vi "Get.vi"(6 "abort (F)":bool, 11 "TagData in":refnum<class "TagData.lvclass">) -> (0 "element":cluster{timestamp[], dbl[]}[](array[cluster]), 1 "sequence":u64, 2 "update":refnum<k4>, 3 "TagData out":refnum<class "TagData.lvclass">, 4 "aborted?":bool)   [LabVIEW 2020, in "Tag-a[.](c(a[.](stamp),a[.](dbl))).lvlib" / "TagData.lvclass"]
uses:
  <extravilib>/ChannelInstances/Tag-a[.](c(a[.](stamp),a[.](dbl)))/TagData.lvclass
  <extravilib>/ChannelInstances/Tag-a[.](c(a[.](stamp),a[.](dbl)))/TagData.lvclass/TagData.ctl
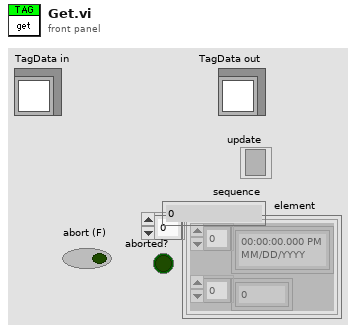
[diagram p1: front panel]
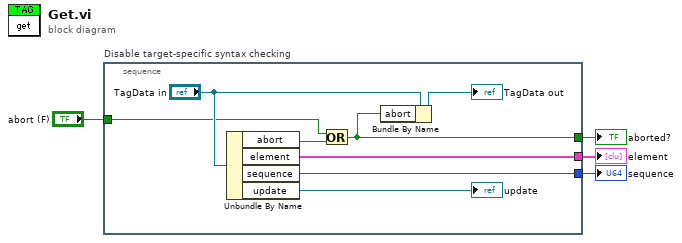
[diagram p0: block diagram]
diagram:
  n1 = stacked-sequence "Disable target-specific syntax checking" {
    tunnel: [w11] -> w4
    tunnel: [w10] -> w3
    tunnel: "abort (F)" -> [w8]
    tunnel: [w5] -> w1
    frame #0 {
      n2 = Unbundle By Name("TagData in") -> ("abort"=w7:bool, "element"=w11:cluster{timestamp[], dbl[]}[], "sequence"=w10:u64, "update"=→"update":refnum<k4>)
      n3 = Or(x=w8, y=w7) -> (x .or. y?=w5:bool)
      n4 = Bundle By Name(cluster="TagData in", "abort"=w5) -> (→"TagData out":refnum<class "TagData.lvclass">)
    }
  }
  "element" <- w4
  "sequence" <- w3
  "aborted?" <- w1
